vi "ReduceFrequenciesToCounts.vi"(1 "Sensor Frequencies (kHz)":dbl[](array[numeric])) -> (0 "Sensor Counts":dbl[](array[numeric]))   [LabVIEW 2013]
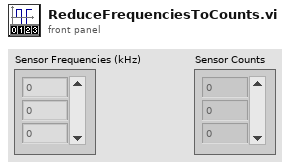
[diagram p1: front panel]
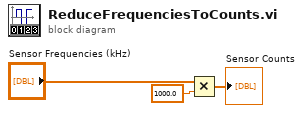
[diagram p0: block diagram]
diagram:
  n1 = Multiply(x="Sensor Frequencies (kHz)", y=1000.0) -> (x*y=→"Sensor Counts":dbl[])
